vi "Reload.vi"(0 "HighRef":T10, 7 "Winch Servo":T1={"DeviceStatus"={"status"=FALSE, "code"=0, "source"=""}, "Digital Module"=enum."Digital Module 1", "PWM Channel"=enum."Invalid", "DeadBand"={"Name"="", "maxPositivePwm"=0, "minPositivePwm"=0, "centerPwm"=0, "maxNegativePwm"=0, "minNegativePwm"=0, "angularRange"=0}}, 11 "ShooterMotorRef":T6={"DeviceStatus"={"status"=FALSE, "code"=0, "source"=""}, "Type"=enum."PWM", "PWM"={"Digital Module"=enum."Digital Module 1", "PWM Channel"=enum."Invalid", "DeadBand"={"Name"="", "maxPositivePwm"=0, "minPositivePwm"=0, "centerPwm"=0, "maxNegativePwm"=0, "minNegativePwm"=0, "angularRange"=0}}, "CAN"={"Device Number"=0, "Control Mode"=enum."Percent VBus", "Semaphore"=refnum, "Max Vout"=12.0}, "Invert"=FALSE, "TransformRef"=refnum, "InvTransformRef"=refnum}) -> (4 "winch engaged?":T5, 10 "Latch engage":bool)   [LabVIEW 2013]
uses:
  <vilib>/Rock Robotics/WPI/Solenoid/WPI_SolenoidValue.ctl
  reload enum.ctl
  <vilib>/Rock Robotics/SystemInterfaces/DIO/FPGA_DIOChannel.ctl
  <vilib>/Rock Robotics/SystemInterfaces/Typedef/FPGA_TypedefDigitalModule.ctl
  <vilib>/Rock Robotics/WPI/DigitalInput/WPI_DigitalInputDevRef.ctl
  <vilib>/Rock Robotics/WPI/PWM/WPI_PWMTransform_ConPane.ctl
  <vilib>/Rock Robotics/SystemInterfaces/DIO/FPGA_DIOPWMChannel.ctl
  <vilib>/Rock Robotics/WPI/PWM/WPI_PWMDeadband.ctl
  <vilib>/Rock Robotics/WPI/CAN/Jaguar/SubVIs/WPI_CANJaguar_ControlMode.ctl
  <vilib>/Rock Robotics/WPI/MotorControl/WPI_MotorControlDeviceRef.ctl
  <vilib>/Rock Robotics/WPI/PWM/Servo/WPI_ServoDeviceRef.ctl
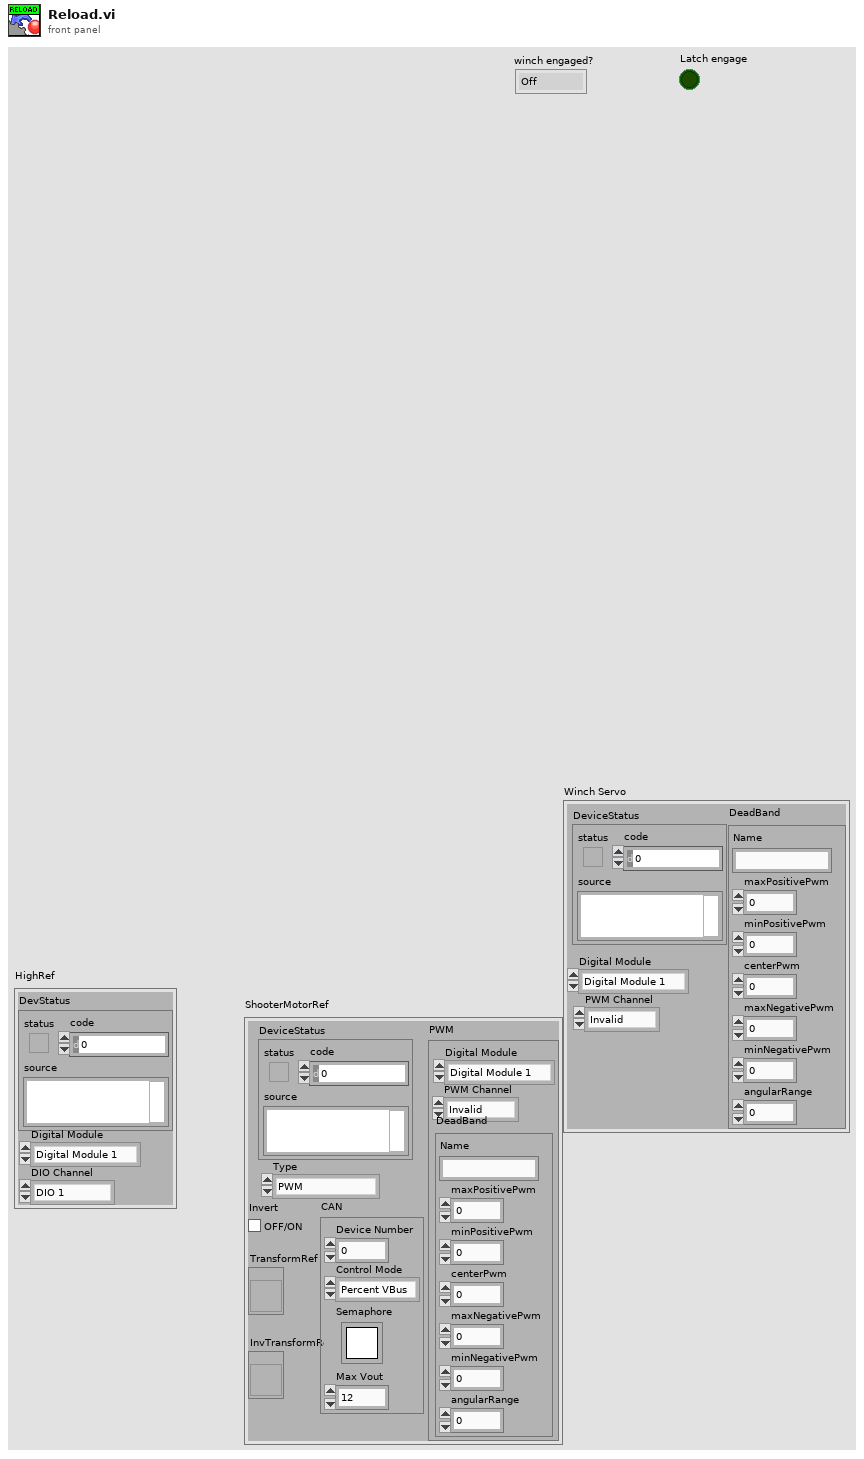
[diagram p1: front panel]
types:
  T1 = typedef "WPI_ServoDeviceRef.ctl" = cluster{"DeviceStatus":errorcluster, "Digital Module":T2, "PWM Channel":T3, "DeadBand":T4}
  T2 = typedef "FPGA_TypedefDigitalModule.ctl" = enum16{"Digital Module 1", "Digital Module 2"}
  T3 = typedef "FPGA_DIOPWMChannel.ctl" = enum8{"PWM 1", "PWM 2", "PWM 3", "PWM 4", "PWM 5", "PWM 6", "PWM 7", "PWM 8", "PWM 9", "PWM 10", "Invalid"}
  T4 = typedef "WPI_PWMDeadband.ctl" = cluster{"Name":string, "maxPositivePwm":i32, "minPositivePwm":i32, "centerPwm":i32, "maxNegativePwm":i32, "minNegativePwm":i32, "angularRange":u16}
  T5 = typedef "WPI_SolenoidValue.ctl" = enum16{"Off", "On", "Forward", "Reverse"}
  T6 = typedef "WPI_MotorControlDeviceRef.ctl" = cluster{"DeviceStatus":errorcluster, "Type":enum16{"PWM", "CAN"}, "PWM":cluster{"Digital Module":T2, "PWM Channel":T3, "DeadBand":T4}, "CAN":cluster{"Device Number":u8, "Control Mode":T7, "Semaphore":T8, "Max Vout":dbl}, "Invert":bool, "TransformRef":T9, "InvTransformRef":T9}
  T7 = typedef "WPI_CANJaguar_ControlMode.ctl" = enum8{"Percent VBus", "Current", "Speed", "Position", "Voltage"}
  T8 = typedef "Semaphore RefNum" = refnum<k1>
  T9 = typedef "WPI_PWMTransform_ConPane.ctl" = refnum<vi>
  T10 = typedef "WPI_DigitalInputDevRef.ctl" = cluster{"DevStatus":errorcluster, "DIO Channel":T11, "Digital Module":T2}
  T11 = typedef "FPGA_DIOChannel.ctl" = enum8{"DIO 1", "DIO 2", "DIO 3", "DIO 4", "DIO 5", "DIO 6", "DIO 7", "DIO 8", "DIO 9", "DIO 10", "DIO 11", "DIO 12", "DIO 13", "DIO 14", "Invalid"}
  T12 = typedef "reload enum.ctl" = enum16{"winch runs", "winch stops", "gearbox release", "gearbox engage", "Wait for shot", "Wait for fire"}
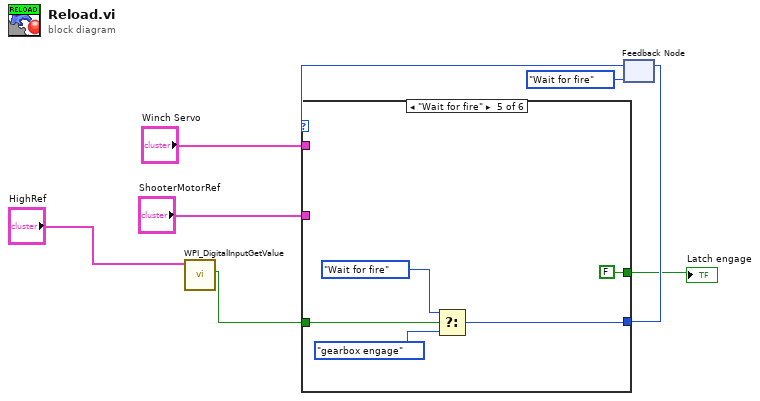
[diagram p0: block diagram]
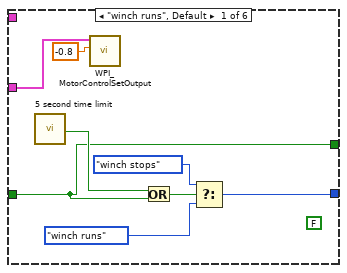
[diagram p2: hidden frame]
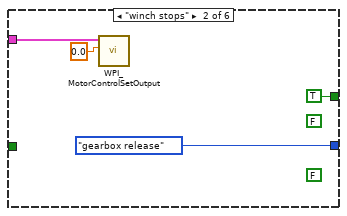
[diagram p3: hidden frame]
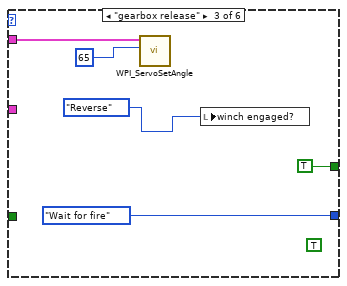
[diagram p4: hidden frame]
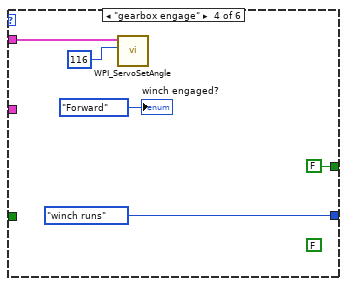
[diagram p5: hidden frame]
diagram:
  n1 = call <vilib>:"WPI_DigitalInputGetValue.vi"("DigitalInputDevRef"="HighRef") -> ("Value"=w1:bool)  [unwired: 8 in, 2 out]
  n2 = feedback #1(reload_enum."Wait for fire") -> (w7:T12)
  n3 = case shown="\"Wait for fire\"" w7 {
    tunnel: [w13 reload_enum."gearbox release" reload_enum."Wait for fire" reload_enum."winch runs" w35 _] -> w8
    tunnel: "ShooterMotorRef" -> [w12 w19 _ _ _ _]
    tunnel: "Winch Servo" -> [_ _ w24 w28 _ _]
    tunnel: [w9 TRUE TRUE FALSE ("Value") FALSE ("Value") _] -> w3
    tunnel: w1 -> [w9 _ _ _ w31 _]
    frame "winch runs", Default {
      (unwired) FALSE ("Value")
      n4 = call "5 second time limit"() -> ("Time has Elapsed"=w11:bool)  [unwired: 12 in, 7 out]
      n5 = call <vilib>:"WPI_MotorControlSetOutput.vi"("Output"=-0.8, "MotorControlDevRef"=w12) -> ()  [unwired: 7 in, 3 out]
      n6 = Or(x=w11, y=w9) -> (x .or. y?=w10:bool)
      n7 = Select(t=reload_enum."winch stops", s=w10, f=reload_enum."winch runs") -> (s? t:f=w13:T12)
    }
    frame "winch stops" {
      (unwired) FALSE
      (unwired) FALSE ("Value")
      n8 = call <vilib>:"WPI_MotorControlSetOutput.vi"("Output"=0.0, "MotorControlDevRef"=w19) -> ()  [unwired: 7 in, 3 out]
    }
    frame "gearbox release" {
      (unwired) TRUE ("Value")
      n9 = call <vilib>:"WPI_ServoSetAngle.vi"("Angle"=65, "ServoDeviceRef"=w24) -> ()  [unwired: 8 in, 2 out]
      n10 = local write "winch engaged?"(WPI_SolenoidValue."Reverse" ("Value")) -> ()
    }
    frame "gearbox engage" {
      (unwired) FALSE ("Value")
      n11 = call <vilib>:"WPI_ServoSetAngle.vi"("Angle"=116, "ServoDeviceRef"=w28) -> ()  [unwired: 8 in, 2 out]
      "winch engaged?" <- WPI_SolenoidValue."Forward" ("Value")
    }
    frame "Wait for fire" {
      n12 = Select(t=reload_enum."Wait for fire", s=w31, f=reload_enum."gearbox engage") -> (s? t:f=w35:T12)
    }
    frame "Wait for shot" {
    }
  }
  "Latch engage" <- w3
  n13 = feedback-in #1(w8) -> ()
